vi "AT_Pass_Or_Fail.vi"(10 "Valor Dado":string, 11 "Valor Esperado":string) -> (1 "Result":string, 2 "Valor esperado":string, 3 "Valor dado":string)   [LabVIEW 2021]
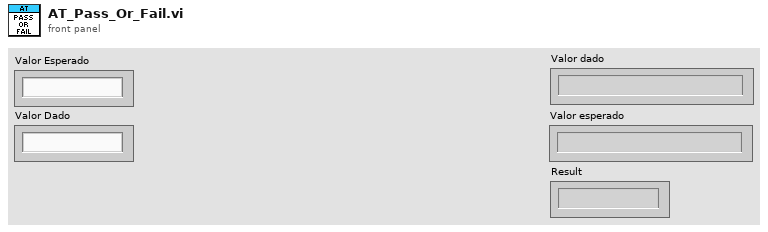
[diagram p1: front panel]
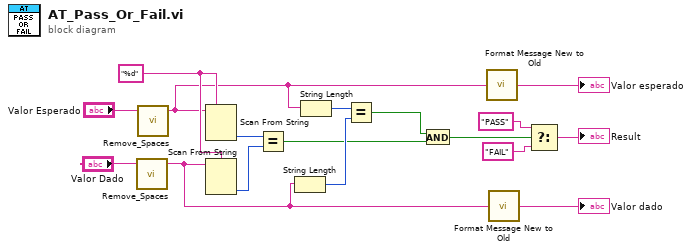
[diagram p0: block diagram]
diagram:
  w17 = "%d" ("format string")
  n1 = call "Remove_Spaces.vi"("input string"="Valor Dado") -> ("result string"=w5:string)  [unwired: 4 in]
  n2 = call "Remove_Spaces.vi"("input string"="Valor Esperado") -> ("result string"=w7:string)  [unwired: 4 in]
  n3 = Scan From String(format string=w17, input string=w7) -> (output 1=w14:i32)  [unwired: 3 in, 3 out]
  n4 = Scan From String(format string=w17, input string=w5) -> (output 1=w13:i32)  [unwired: 3 in, 3 out]
  n5 = Equal?(x=w14, y=w13) -> (x = y?=w3:bool)
  n6 = String Length(string=w5) -> (length=w4:i32)
  n7 = String Length(string=w7) -> (length=w6:i32)
  n8 = Equal?(x=w6, y=w4) -> (x = y?=w2:bool)
  n9 = And(x=w2, y=w3) -> (x .and. y?=w1:bool)
  n10 = call "Format Message New to Old.vi"("Raw Message In"=w7) -> ("Conv Message Out"=→"Valor esperado":string)  [unwired: 14 in]
  n11 = call "Format Message New to Old.vi"("Raw Message In"=w5) -> ("Conv Message Out"=→"Valor dado":string)  [unwired: 14 in]
  n12 = Select(t="PASS" ("String"), s=w1, f="FAIL") -> (s? t:f=→"Result":string)
